vi "Initialize.vi"(8 "error in (no error)":errorcluster, 9 "Reset (True)":bool=TRUE, 10 "ID Query (True)":bool=TRUE, 11 "VISA resource name":refnum<visa-resource-name>) -> (0 "error out":errorcluster, 3 "VISA resource name out":refnum<visa-resource-name>)   [LabVIEW 2012, in "Agilent 8000 Series.lvlib"]
doc: "Establishes communication with the instrument and optionally performs an instrument identification query and/or an instrument reset. It also places the instrument in a default state needed for other instrument driver operations. Therefore, call this VI before calling other instrument driver VIs for this instrument. Generally, you need to call the Initialize VI only once at the beginning of an application."
uses:
  Agilent 8000 Series.lvlib
  <vilib>/regexp/Match Regular Expression.xnode
panel:
  # "(c) 2008-2015 National Instruments.  ALL RIGHTS RESERVED."
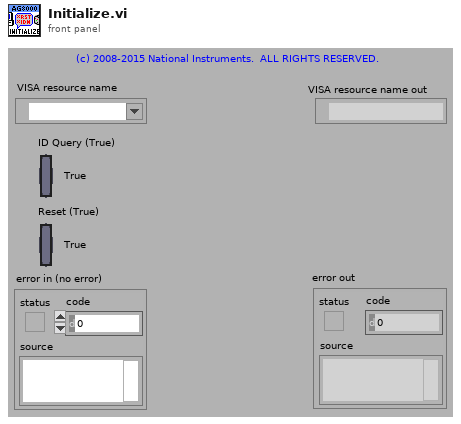
[diagram p1: front panel]
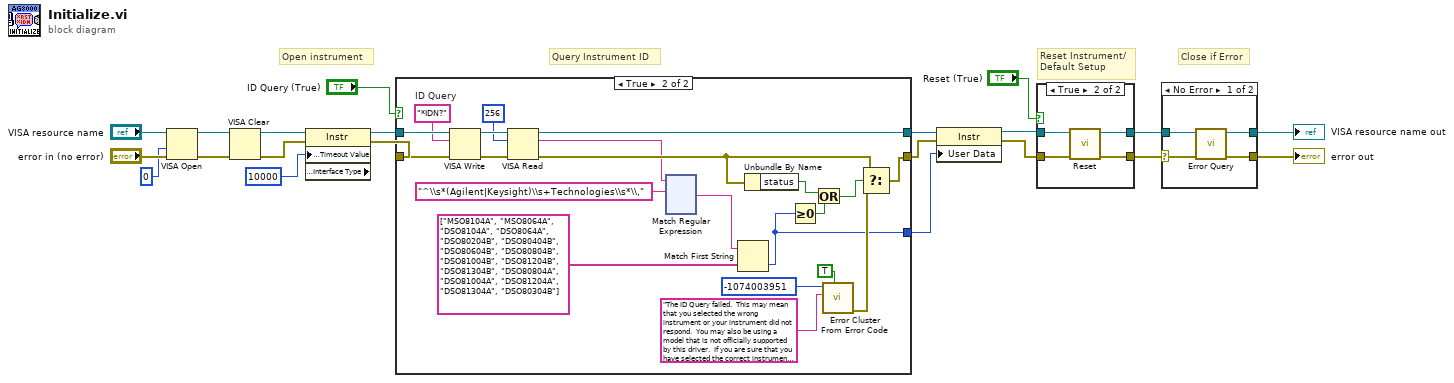
[diagram p0: block diagram]
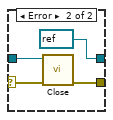
[diagram p2: hidden frame]
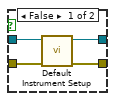
[diagram p3: hidden frame]
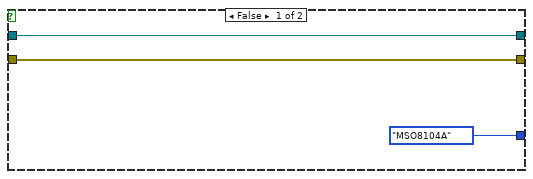
[diagram p4: hidden frame]
diagram:
  # "Close if Error"
  # "Query Instrument ID"
  # "Reset Instrument/\nDefault Setup"
  # "Open instrument"
  n1 = VISA Open(access mode=u32 0, error in (no error)="error in (no error)", VISA resource name="VISA resource name") -> (VISA resource name=w15:refnum<visa-resource-name>, error out=w14:errorcluster)  [unwired: 2 in]
  n2 = VISA Clear(VISA resource name=w15, error in (no error)=w14) -> (VISA resource name out=w13:refnum<visa-resource-name>, error out=w12:errorcluster)
  n3 = property class="Instr" props=["General Settings:Timeout Value", "Interface Information:Interface Type"](reference=w13, error in=w12, "General Settings:Timeout Value"=u32 10000) -> (reference out=w7:refnum<visa-resource-name>, error out=w6:errorcluster)  [unwired: 1 out]
  n4 = case shown="True" "ID Query (True)" {
    tunnel: [w23 w29] -> w5
    tunnel: [w24 w43] -> w4
    tunnel: w7 -> [w24 w44]
    tunnel: w6 -> [w23 w45]
    tunnel: [enum16{"MSO8104A"}."MSO8104A" w28] -> w1
    frame False {
    }
    frame True {
      w39 = "*IDN?"  # ID Query
      n5 = VISA Write(VISA resource name=w44, write buffer=w39, error in (no error)=w45) -> (VISA resource name out=w42:refnum<visa-resource-name>, error out=w41:errorcluster)  [unwired: 1 out]
      n6 = VISA Read(VISA resource name=w42, byte count=u32 256, error in (no error)=w41) -> (VISA resource name out=w43:refnum<visa-resource-name>, read buffer=w27:string, error out=w34:errorcluster)  [unwired: 1 out]
      n7 = xnode ("Match Regular Expression")("input string"=w27, "regular expression"="^\\s*(Agilent|Keysight)\\s+Technologies\\s*\\," ("Company Name Regular Expression")) -> ("after match"=w25:string)  [unwired: 4 in, 4 out]
      n8 = Match First String(2:string[] ["MSO8104A", "MSO8064A", "DSO8104A", "DSO8064A", "DSO80204B", "DSO80404B", "DSO80604B", "DSO80804B", "DSO81004B", "DSO81204B", "DSO81304B", "DSO80804A", "DSO81004A", "DSO81204A", "DSO81304A", "DSO80304B"], 3:w25) -> (0:w28:i32)  [unwired: 1 out]
      n9 = Unbundle By Name(w34) -> ("status"=w33:bool)
      n10 = Greater Or Equal To 0?(x=w28) -> (x >= 0?=w32:bool)
      n11 = Or(x=w33, y=w32) -> (x .or. y?=w31:bool)
      n12 = call <vilib>:"Error Cluster From Error Code.vi"("show call chain? (False)"=TRUE, "error message (\"\")"="The ID Query failed.  This may mean that you selected the wrong instrument or your instrument did not respond.  You may also be using a model that is not officially supported by this driver.  If you are sure that you have selected the correct instrument and it is responding, try disabling the ID Query." ("Source (VI Name)"), "error code (0)"=-1074003951 ("Code")) -> ("error out"=w38:errorcluster)  [unwired: 6 in]
      n13 = Select(t=w34, s=w31, f=w38) -> (s? t:f=w29:errorcluster)
    }
  }
  n14 = property class="Instr"(reference=w4, error in=w5, "User Data"=w1) -> (reference out=w3:refnum<visa-resource-name>, error out=w2:errorcluster)
  n15 = case shown="True" "Reset (True)" {
    tunnel: w2 -> [w159 w161]
    tunnel: [w158 w164] -> w8
    tunnel: w3 -> [w160 w162]
    tunnel: [w157 w163] -> w9
    frame False {
      n16 = call "Default Instrument Setup.vi"("error in (no error)"=w159, "VISA resource name"=w160) -> ("error out"=w158:errorcluster, "VISA resource name out"=w157:refnum<visa-resource-name>)  [unwired: 8 in]
    }
    frame True {
      n17 = call "Reset.vi"("error in (no error)"=w161, "VISA resource name"=w162) -> ("error out"=w164:errorcluster, "VISA resource name out"=w163:refnum<visa-resource-name>)  [unwired: 8 in]
    }
  }
  n18 = case shown="No Error" w8 {
    selector: w8 -> [w166 w170]
    tunnel: w9 -> [w165 w171]
    tunnel: [w168 refnum<visa-resource-name> refnum ("VISA resource name out")] -> w11
    tunnel: [w167 w172] -> w10
    frame No Error {
      n19 = call "Error Query.vi"("error in (no error)"=w166, "VISA resource name"=w165) -> ("error out"=w167:errorcluster, "VISA resource name out"=w168:refnum<visa-resource-name>)  [unwired: 6 in, 2 out]
    }
    frame Error {
      n20 = call <instrlib>:"Close.vi"("error in (no error)"=w170, "VISA resource name"=w171) -> ("error out"=w172:errorcluster)  [unwired: 9 in]
    }
  }
  "VISA resource name out" <- w11
  "error out" <- w10
